vi "Testing Functional Test.vi"(7 "FrequencyCounter":refnum<visa-resource-name>, 8 "connection information":path, 9 "System Number":string, 10 "error in":errorcluster, 11 "Arduino":refnum<visa-resource-name>) -> (1 "Functional Test Data":string, 2 "error out":errorcluster, 3 "Arduino":refnum<visa-resource-name>)   [LabVIEW 2024]
uses:
  <vilib>/addons/database/Connection.llb/DB Tools Open Connec (Path).vi
  Agilent 532XX Series/Public/Configure/Measurement/Configure Measurement (Frequency).vi
  <vilib>/addons/database/_DB Variant To Data/Database Variant To Data.xnode
  <vilib>/addons/database/NI_Database_API.lvlib
  Agilent 532XX Series/Agilent 532XX Series.lvlib
panel:
  out "Command Array":string[](array[string])
  out "Upper Position":i32
  out "Lower Position":i32
  out "Functional Test Data Rack 2":string
  out "Functional Test Data Rack 1":string
  out "Lower Rack":dbl
  out "Upper Rack":dbl
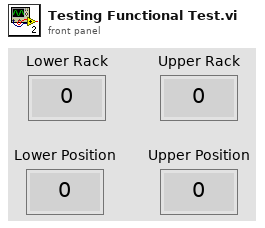
[diagram p1: front panel]
types:
  T1 = typedef "NI_Database_API.lvlib/Conn ObjectReference.ctl" = refnum<k1>
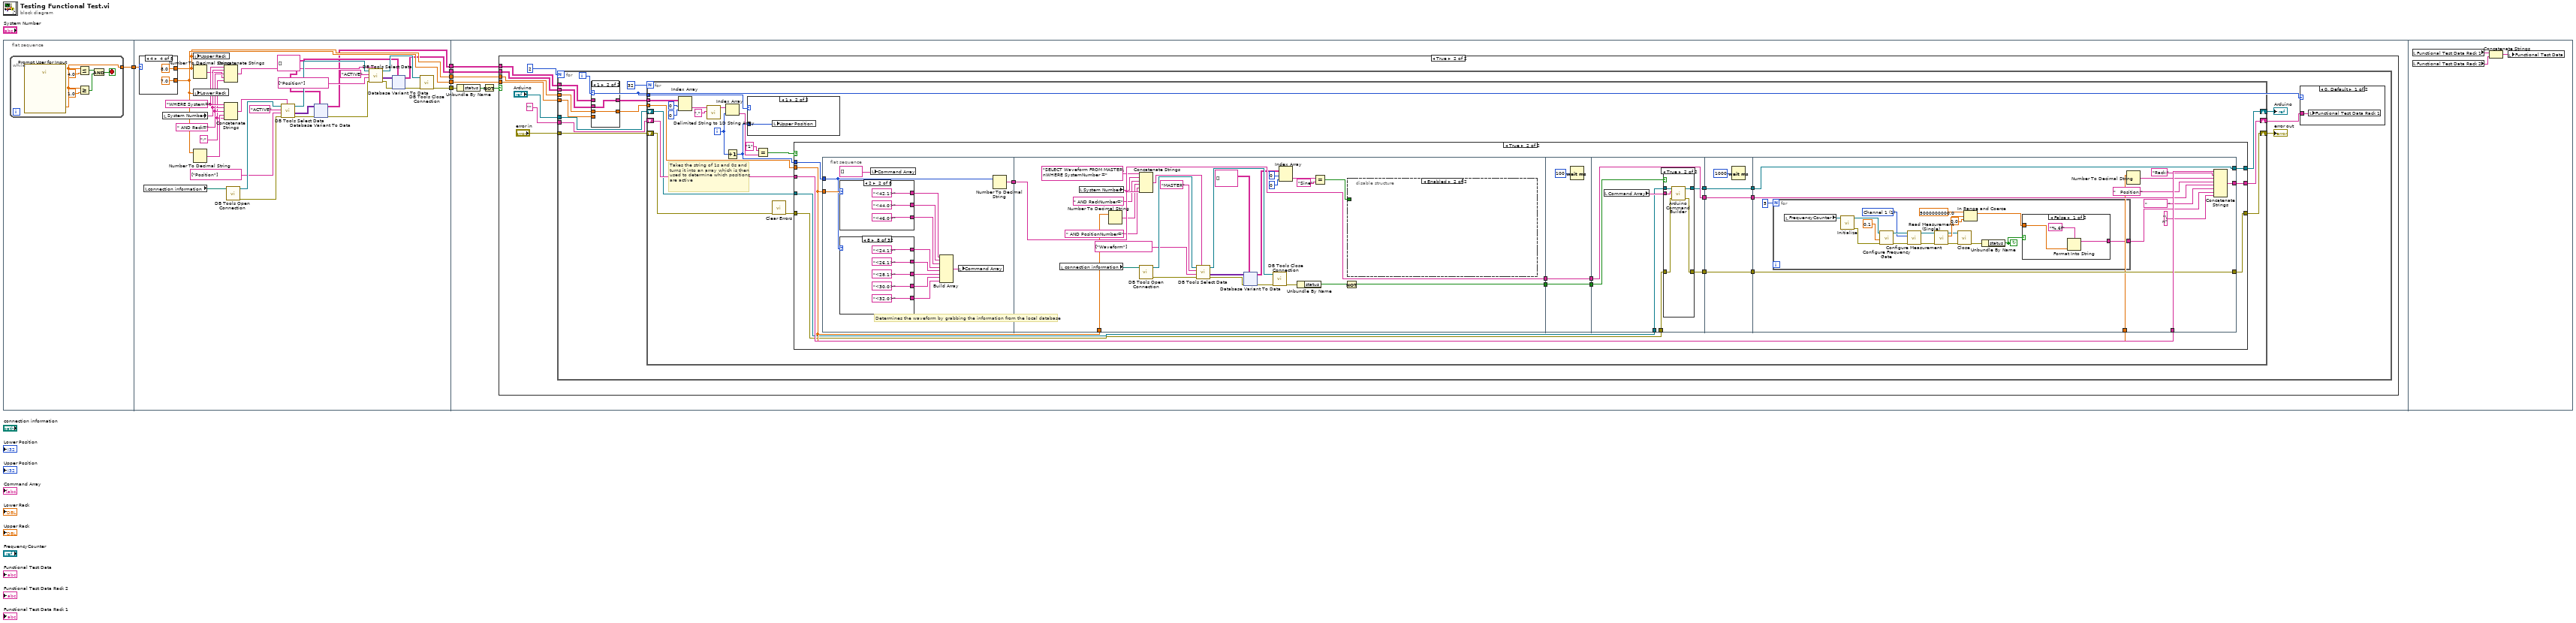
[diagram p0: block diagram]
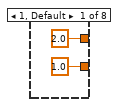
[diagram p2: hidden frame]
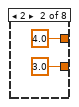
[diagram p3: hidden frame]
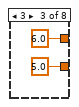
[diagram p4: hidden frame]
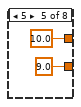
[diagram p5: hidden frame]
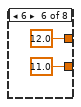
[diagram p6: hidden frame]
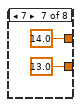
[diagram p7: hidden frame]
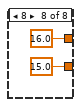
[diagram p8: hidden frame]
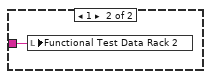
[diagram p10: hidden frame]
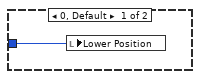
[diagram p12: hidden frame]
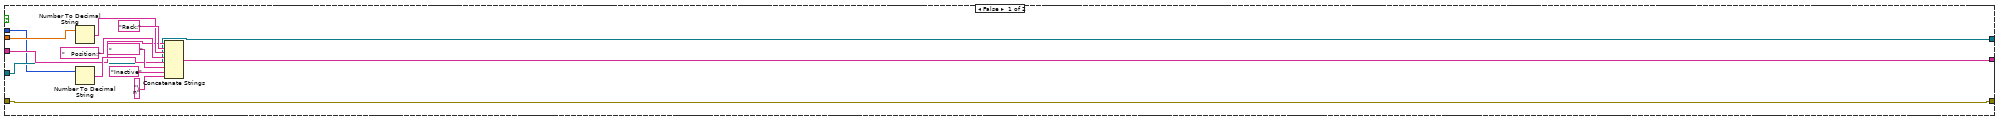
[diagram p13: hidden frame]
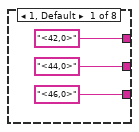
[diagram p14: hidden frame]
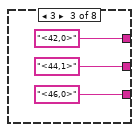
[diagram p15: hidden frame]
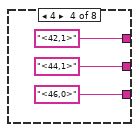
[diagram p16: hidden frame]
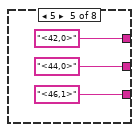
[diagram p17: hidden frame]
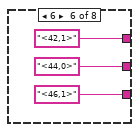
[diagram p18: hidden frame]
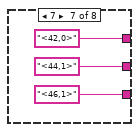
[diagram p19: hidden frame]
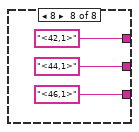
[diagram p20: hidden frame]
diagram:
  n1 = flat-sequence {
    tunnel: [w7] -> w2
    tunnel: [w16] -> w6
    tunnel: [w15] -> w5
    tunnel: [w36] -> w4
    tunnel: [w38] -> w3
    tunnel: w2 -> [w35]
    tunnel: [w30] -> w1
    tunnel: w3 -> [w153]
    tunnel: w4 -> [w154]
    tunnel: w5 -> [w151]
    tunnel: w6 -> [w152]
    tunnel: w1 -> [w148]
    frame #0 {
      n2 = while {
        tunnel: [w13] -> w7
        stop <- w10 stop-if-true
        n3 = call "Prompt User for Input"() -> ("Shelf Number"=w13:dbl)  [unwired: 17 in, 2 out]
        n4 = Less Or Equal?(x=w13, y=4.0) -> (x <= y?=w9:bool)
        n5 = Greater Or Equal?(x=w13, y=1.0) -> (x >= y?=w8:bool)
        n6 = And(x=w9, y=w8) -> (x .and. y?=w10:bool)
      }
    }
    frame #1 {
      w18 = string[][] []
      w41 = " AND Rack="
      w39 = ";" ("string")
      w42 = "WHERE System=" ("SQL Query")
      n7 = case shown="4" w35 {
        tunnel: [1.0 ("y") 3.0 ("y") 5.0 ("y") 7.0 ("y") 9.0 ("y") 11.0 ("y") 13.0 ("y") 15.0 ("y")] -> w38
        tunnel: [2.0 ("y") 4.0 ("y") 6.0 ("y") 8.0 ("y") 10.0 ("y") 12.0 ("y") 14.0 ("y") 16.0 ("y")] -> w36
        frame 1, Default {
        }
        frame 2 {
        }
        frame 3 {
        }
        frame 4 {
        }
        frame 5 {
        }
        frame 6 {
        }
        frame 7 {
        }
        frame 8 {
        }
      }
      n8 = local read "connection information"() -> (w14:path)
      n9 = local read "System Number"() -> (w40:string)
      n10 = local write "Upper Rack"(w36) -> ()
      n11 = Number To Decimal String(number=w36) -> (decimal integer string=w37:string)  [unwired: 1 in]
      n12 = local write "Lower Rack"(w38) -> ()
      n13 = Number To Decimal String(number=w38) -> (decimal integer string=w43:string)  [unwired: 1 in]
      n14 = Concatenate Strings(w42, w40, w41, w37, w39) -> (w21:string)
      n15 = Concatenate Strings(w42, w40, w41, w43, w39) -> (w20:string)
      n16 = call-poly <vilib>:"DB Tools Open Connection.vi"("connection information"=w14) -> ("error out"=w29:errorcluster, "connection reference"=w28:T1)  [unwired: 7 in]
      n17 = call <vilib>:"DB Tools Select Data.vi"("condition"=w20, "error in (no error)"=w29, "columns"=string[] ["Position"], "table"="ACTIVE", "connection reference"=w28) -> ("error out"=w34:errorcluster, "data"=w17:variant[][], "connection reference out"=w27:T1)  [unwired: 1 in]
      n18 = xnode "Database Variant To Data"("database variant"=w17, "error in (no error)"=w34, "type"=w18) -> ("data"=w16:string[][], "error out"=w33:errorcluster)
      n19 = call <vilib>:"DB Tools Select Data.vi"("condition"=w21, "error in (no error)"=w33, "columns"=string[] ["Position"], "table"="ACTIVE", "connection reference"=w27) -> ("error out"=w32:errorcluster, "data"=w19:variant[][], "connection reference out"=w26:T1)  [unwired: 1 in]
      n20 = xnode "Database Variant To Data"("database variant"=w19, "error in (no error)"=w32, "type"=w18) -> ("data"=w15:string[][], "error out"=w31:errorcluster)
      n21 = call <vilib>:"DB Tools Close Connection.vi"("error in (no error)"=w31, "connection reference"=w26) -> ("error out"=w30:errorcluster)  [unwired: 5 in]
    }
    frame #2 {
      n22 = Unbundle By Name(w148) -> ("status"=w150:bool)
      n23 = Not(x=w150) -> (.not. x?=w149:bool)
      n24 = case shown="True" w149 {
        tunnel: w154 -> [_ w158]
        tunnel: w153 -> [_ w157]
        tunnel: w152 -> [_ w156]
        tunnel: w151 -> [_ w155]
        frame False {
        }
        frame True {
          n25 = for {
            N: 2 -> [_]
            tunnel: "" -> [w176]
            tunnel: w156 -> [w172]
            tunnel: "error in" -> [w174]
            tunnel: "Arduino" -> [w173]
            tunnel: w155 -> [w171]
            tunnel: w158 -> [w169]
            tunnel: w157 -> [w168]
            i -> [w165]
            n26 = case shown="1" w165 {
              tunnel: w172 -> [w180 _]
              tunnel: w171 -> [_ w182]
              tunnel: [w180 w182] -> w170
              tunnel: w169 -> [_ w181]
              tunnel: w168 -> [w179 _]
              tunnel: [w179 w181] -> w167
              frame 0, Default {
              }
              frame 1 {
              }
            }
            n27 = for {
              N: 32 -> [_]
              shift-right: [w191] -> w166
              shift-left: w176 -> [w192]
              tunnel: w167 -> [w193]
              tunnel: w170 -> [w197]
              shift-right: [w189] -> w164
              shift-left: w173 -> [w184]
              shift-right: [w190] -> w163
              shift-left: w174 -> [w202]
              tunnel: w165 -> [w185]
              i -> [w187]
              # "Takes the string of 1s and 0s and turns it into an array which is then used to determine which positions are active"
              n28 = Index Array(array=w197, index (row)=0 ("disabled index (row)"), index (col)=0 ("disabled index (col)")) -> (element=w199:string)
              n29 = call <vilib>:"Delimited String to 1D String Array.vi"("delimiter"=",", "delimited string"=w199) -> ("string array"=w200:string[])  [unwired: 9 in]
              n30 = Index Array(array=w200, index=w187) -> (element=w201:string)
              n31 = Increment(x=w187) -> (x+1=w186:i32)
              n32 = case shown="1" w185 {
                tunnel: w186 -> [w203 w204]
                frame 0, Default {
                  n33 = local write "Lower Position"(w203) -> ()
                }
                frame 1 {
                  n34 = local write "Upper Position"(w204) -> ()
                }
              }
              n35 = Equal?(x="1", y=w201) -> (x = y?=w188:bool)
              n36 = call <vilib>:"Clear Errors.vi"("error in (no error)"=w202) -> ("error out"=w183:errorcluster)  [unwired: 5 in, 1 out]
              n37 = case shown="True" w188 {
                tunnel: w186 -> [w205 w236]
                tunnel: w193 -> [w208 w230]
                tunnel: w192 -> [w209 w235]
                tunnel: w184 -> [w206 w220]
                tunnel: w183 -> [w207 w225]
                tunnel: [w211 w234] -> w191
                tunnel: [w207 w233] -> w190
                tunnel: [w206 w232] -> w189
                frame False {
                  n38 = Number To Decimal String(number=w208) -> (decimal integer string=w216:string)  [unwired: 1 in]
                  n39 = Number To Decimal String(number=w205) -> (decimal integer string=w210:string)  [unwired: 1 in]
                  n40 = Concatenate Strings(w209, "Rack:" ("string"), w216, "   Position:" ("string"), w210, "              " ("string"), "Inactive" ("string"), "\n" ("string")) -> (w211:string)
                }
                frame True {
                  n41 = flat-sequence {
                    tunnel: [w249] -> w231
                    tunnel: w236 -> [w247]
                    tunnel: w230 -> [w248]
                    tunnel: w231 -> [w460]
                    tunnel: [w460] -> w229
                    tunnel: w230 -> [w452]
                    tunnel: [w447] -> w218
                    tunnel: w229 -> [w520]
                    tunnel: [w520] -> w228
                    tunnel: [w518] -> w219
                    tunnel: w218 -> [w518]
                    tunnel: w228 -> [w527]
                    tunnel: [w527] -> w227
                    tunnel: w225 -> [w525]
                    tunnel: [w524] -> w223
                    tunnel: [w523] -> w221
                    tunnel: w220 -> [w522]
                    tunnel: w219 -> [w521]
                    tunnel: w227 -> [w538]
                    tunnel: [w538] -> w226
                    tunnel: [w536] -> w224
                    tunnel: w223 -> [w536]
                    tunnel: [w535] -> w222
                    tunnel: w221 -> [w535]
                    tunnel: w235 -> [w551]
                    tunnel: w230 -> [w541]
                    tunnel: [w550] -> w234
                    tunnel: [w543] -> w233
                    tunnel: [w542] -> w232
                    tunnel: w226 -> [w549]
                    tunnel: w224 -> [w543]
                    tunnel: w222 -> [w542]
                    frame #0 {
                      # "Determines the waveform by grabbing the information from the local database"
                      n42 = case shown="2" w248 {
                        tunnel: ["<42,0>" ("string") "<42,1>" ("string") "<42,0>" ("string") "<42,1>" ("string") "<42,0>" ("string") "<42,1>" ("string") "<42,0>" ("string") "<42,1>" ("string")] -> w240
                        tunnel: ["<44,0>" ("string") "<44,0>" ("string") "<44,1>" ("string") "<44,1>" ("string") "<44,0>" ("string") "<44,0>" ("string") "<44,1>" ("string") "<44,1>" ("string")] -> w239
                        tunnel: ["<46,0>" ("string") "<46,0>" ("string") "<46,0>" ("string") "<46,0>" ("string") "<46,1>" ("string") "<46,1>" ("string") "<46,1>" ("string") "<46,1>" ("string")] -> w238
                        frame 1, Default {
                        }
                        frame 2 {
                        }
                        frame 3 {
                        }
                        frame 4 {
                        }
                        frame 5 {
                        }
                        frame 6 {
                        }
                        frame 7 {
                        }
                        frame 8 {
                        }
                      }
                      n43 = case shown="8" w247 {
                        tunnel: ["<32,0>" ("string") "<32,0>" ("string") "<32,0>" ("string") "<32,0>" ("string") "<32,0>" ("string") "<32,0>" ("string") "<32,0>" ("string") "<32,0>" ("string") "<32,0>" ("string") "<32,0>" ("string") "<32,0>" ("string") "<32,0>" ("string") "<32,0>" ("string") "<32,0>" ("string") "<32,0>" ("string") "<32,0>" ("string") "<32,1>" ("string") "<32,1>" ("string") "<32,1>" ("string") "<32,1>" ("string") "<32,1>" ("string") "<32,1>" ("string") "<32,1>" ("string") "<32,1>" ("string") "<32,1>" ("string") "<32,1>" ("string") "<32,1>" ("string") "<32,1>" ("string") "<32,1>" ("string") "<32,1>" ("string") "<32,1>" ("string") "<32,1>" ("string")] -> w242
                        tunnel: ["<30,0>" ("string") "<30,0>" ("string") "<30,0>" ("string") "<30,0>" ("string") "<30,0>" ("string") "<30,0>" ("string") "<30,0>" ("string") "<30,0>" ("string") "<30,1>" ("string") "<30,1>" ("string") "<30,1>" ("string") "<30,1>" ("string") "<30,1>" ("string") "<30,1>" ("string") "<30,1>" ("string") "<30,1>" ("string") "<30,0>" ("string") "<30,0>" ("string") "<30,0>" ("string") "<30,0>" ("string") "<30,0>" ("string") "<30,0>" ("string") "<30,0>" ("string") "<30,0>" ("string") "<30,1>" ("string") "<30,1>" ("string") "<30,1>" ("string") "<30,1>" ("string") "<30,1>" ("string") "<30,1>" ("string") "<30,1>" ("string") "<30,1>" ("string")] -> w243
                        tunnel: ["<28,0>" ("string") "<28,0>" ("string") "<28,0>" ("string") "<28,0>" ("string") "<28,1>" ("string") "<28,1>" ("string") "<28,1>" ("string") "<28,1>" ("string") "<28,0>" ("string") "<28,0>" ("string") "<28,0>" ("string") "<28,0>" ("string") "<28,1>" ("string") "<28,1>" ("string") "<28,1>" ("string") "<28,1>" ("string") "<28,0>" ("string") "<28,0>" ("string") "<28,0>" ("string") "<28,0>" ("string") "<28,1>" ("string") "<28,1>" ("string") "<28,1>" ("string") "<28,1>" ("string") "<28,0>" ("string") "<28,0>" ("string") "<28,0>" ("string") "<28,0>" ("string") "<28,1>" ("string") "<28,1>" ("string") "<28,1>" ("string") "<28,1>" ("string")] -> w244
                        tunnel: ["<26,0>" ("string") "<26,0>" ("string") "<26,1>" ("string") "<26,1>" ("string") "<26,0>" ("string") "<26,0>" ("string") "<26,1>" ("string") "<26,1>" ("string") "<26,0>" ("string") "<26,0>" ("string") "<26,1>" ("string") "<26,1>" ("string") "<26,0>" ("string") "<26,0>" ("string") "<26,1>" ("string") "<26,1>" ("string") "<26,0>" ("string") "<26,0>" ("string") "<26,1>" ("string") "<26,1>" ("string") "<26,0>" ("string") "<26,0>" ("string") "<26,1>" ("string") "<26,1>" ("string") "<26,0>" ("string") "<26,0>" ("string") "<26,1>" ("string") "<26,1>" ("string") "<26,0>" ("string") "<26,0>" ("string") "<26,1>" ("string") "<26,1>" ("string")] -> w245
                        tunnel: ["<24,0>" ("string") "<24,1>" ("string") "<24,0>" ("string") "<24,1>" ("string") "<24,0>" ("string") "<24,1>" ("string") "<24,0>" ("string") "<24,1>" ("string") "<24,0>" ("string") "<24,1>" ("string") "<24,0>" ("string") "<24,1>" ("string") "<24,0>" ("string") "<24,1>" ("string") "<24,0>" ("string") "<24,1>" ("string") "<24,0>" ("string") "<24,1>" ("string") "<24,0>" ("string") "<24,1>" ("string") "<24,0>" ("string") "<24,1>" ("string") "<24,0>" ("string") "<24,1>" ("string") "<24,0>" ("string") "<24,1>" ("string") "<24,0>" ("string") "<24,1>" ("string") "<24,0>" ("string") "<24,1>" ("string") "<24,0>" ("string") "<24,1>" ("string")] -> w246
                        frame 1, Default {
                        }
                        frame 2 {
                        }
                        frame 3 {
                        }
                        frame 4 {
                        }
                        frame 5 {
                        }
                        frame 6 {
                        }
                        frame 7 {
                        }
                        frame 8 {
                        }
                        frame 9 {
                        }
                        frame 10 {
                        }
                        frame 11 {
                        }
                        frame 12 {
                        }
                        frame 13 {
                        }
                        frame 14 {
                        }
                        frame 15 {
                        }
                        frame 16 {
                        }
                        frame 17 {
                        }
                        frame 18 {
                        }
                        frame 19 {
                        }
                        frame 20 {
                        }
                        frame 21 {
                        }
                        frame 22 {
                        }
                        frame 23 {
                        }
                        frame 24 {
                        }
                        frame 25 {
                        }
                        frame 26 {
                        }
                        frame 27 {
                        }
                        frame 28 {
                        }
                        frame 29 {
                        }
                        frame 30 {
                        }
                        frame 31 {
                        }
                        frame 32 {
                        }
                      }
                      n44 = local write "Command Array"(string[] [] ("Command Array")) -> ()
                      n45 = Build Array(w240, w239, w238, w246, w245, w244, w243, w242) -> (w241:string[])
                      n46 = local write "Command Array"(w241) -> ()
                      n47 = Number To Decimal String(number=w247) -> (decimal integer string=w249:string)  [unwired: 1 in]
                    }
                    frame #1 {
                      n48 = local read "connection information"() -> (w444:path)
                      n49 = local read "System Number"() -> (w457:string)
                      n50 = Number To Decimal String(number=w452) -> (decimal integer string=w458:string)  [unwired: 1 in]
                      n51 = Concatenate Strings("SELECT Waveform FROM MASTER\nWHERE SystemNumber =" ("SQL Query"), w457, " AND RackNumber=" ("string"), w458, " AND PositionNumber=" ("string"), w460) -> (w441:string)
                      n52 = call-poly <vilib>:"DB Tools Open Connection.vi"("connection information"=w444) -> ("error out"=w445:errorcluster, "connection reference"=w443:T1)  [unwired: 7 in]
                      n53 = call <vilib>:"DB Tools Select Data.vi"("condition"=w441, "error in (no error)"=w445, "columns"=string[] ["Waveform"], "table"="MASTER", "connection reference"=w443) -> ("error out"=w446:errorcluster, "data"=w435:variant[][], "connection reference out"=w439:T1)  [unwired: 1 in]
                      n54 = xnode "Database Variant To Data"("database variant"=w435, "error in (no error)"=w446, "type"=string[][] []) -> ("data"=w437:string[][], "error out"=w438:errorcluster)
                      n55 = call <vilib>:"DB Tools Close Connection.vi"("error in (no error)"=w438, "connection reference"=w439) -> ("error out"=w434:errorcluster)  [unwired: 5 in]
                      n56 = Index Array(array=w437, index (row)=0, index (col)=0) -> (element=w459:string)
                      n57 = Unbundle By Name(w434) -> ("status"=w448:bool)
                      n58 = Equal?(x=w459, y="Sine") -> (x = y?=w456:bool)
                      n59 = Not(x=w448) -> (.not. x?=w447:bool)
                      n60 = disable-structure shown="Enabled" {
                        disable-tunnel: w456 -> [w461 _]
                        frame Disabled {
                          n61 = case shown="True" w461 {
                            frame False {
                              n62 = flat-sequence {
                                frame #0 {
                                n63 = Send(0:0 ("bus"), 2:i16 3 ("address"), 5:"INP:COUP DC " ("data string")) -> ()  [unwired: 2 in, 3 out]
                                }
                                frame #1 {
                                n64 = Send(0:0 ("bus"), 2:i16 3 ("address"), 5:"INP:IMP 1.0E6" ("data string")) -> ()  [unwired: 2 in, 3 out]
                                }
                              }
                            }
                            frame True {
                              n65 = flat-sequence {
                                frame #0 {
                                n66 = Send(0:0 ("bus"), 2:i16 3 ("address"), 5:"INP:COUP AC " ("data string")) -> ()  [unwired: 2 in, 3 out]
                                }
                                frame #1 {
                                n67 = Send(0:0 ("bus"), 2:i16 3 ("address"), 5:"INP:IMP 50" ("data string")) -> ()  [unwired: 2 in, 3 out]
                                }
                              }
                            }
                          }
                        }
                        frame Enabled {
                        }
                      }
                    }
                    frame #2 {
                      n68 = Wait (ms)(milliseconds to wait=u32 100) -> ()  [unwired: 1 out]
                    }
                    frame #3 {
                      n69 = local read "Command Array"() -> (w526:string[])
                      n70 = case shown="True" w521 {
                        tunnel: w526 -> [_ w534]
                        tunnel: w525 -> [w528 w533]
                        tunnel: [w528 w532] -> w524
                        tunnel: [w529 w531] -> w523
                        tunnel: w522 -> [w529 w530]
                        frame False {
                        }
                        frame True {
                          n71 = call "Arduino Command Builder.vi"("error in"=w533, "Commands"=w534, "Arduino in"=w530) -> ("error out"=w532:errorcluster, "Arduino out"=w531:refnum<visa-resource-name>)  [unwired: 7 in]
                        }
                      }
                    }
                    frame #4 {
                      n72 = Wait (ms)(milliseconds to wait=u32 1000) -> ()  [unwired: 1 out]
                    }
                    frame #5 {
                      n73 = for {
                        N: 5 -> [_]
                        tunnel: [w552] -> w544
                        stop <- w553 continue-if-true
                        w557 = 1 items=["Channel 1"=1, "Channel 2"=2, "Channel 3"=3] ("Channel (1:Channel 1)")
                        n74 = local read "FrequencyCounter"() -> (w564:refnum<visa-resource-name>)
                        n75 = call "Initialize.vi"("VISA resource name"=w564) -> ("error out"=w559:errorcluster, "VISA resource name out"=w558:refnum<visa-resource-name>)  [unwired: 9 in]
                        n76 = call "Configure Frequency Gate.vi"("error in (no error)"=w559, "Time Resolution (0.1 s)"=0.1 ("number"), "VISA resource name"=w558) -> ("error out"=w568:errorcluster, "VISA resource name out"=w565:refnum<visa-resource-name>)  [unwired: 7 in]
                        n77 = call-poly "Configure Measurement.vi"("error in (no error)"=w568, "Channel (1:Channel 1)"=w557, "VISA resource name"=w565) -> ("error out"=w567:errorcluster, "VISA resource name out"=w566:refnum<visa-resource-name>)  [unwired: 2 in, 5 out]
                        n78 = call "Read Measurement (Single).vi"("error in (no error)"=w567, "VISA resource name"=w566) -> ("error out"=w561:errorcluster, "Measurement"=w562:dbl, "VISA resource name out"=w560:refnum<visa-resource-name>)  [unwired: 7 in]
                        n79 = call "Close.vi"("error in (no error)"=w561, "VISA resource name"=w560) -> ("error out"=w563:errorcluster)  [unwired: 9 in]
                        n80 = In Range and Coerce(upper limit=5000000000.0, x=w562, lower limit=0.0) -> (coerced(x)=w569:dbl)  [unwired: 1 out]
                        n81 = Unbundle By Name(w563) -> ("status"=w553:bool)
                        n82 = case shown="False" w553 {
                          tunnel: [w570 "N/A"] -> w552
                          tunnel: w569 -> [w571 _]
                          frame False {
                            n83 = Format Into String(format string="%.6f", w571) -> (resulting string=w570:string)  [unwired: 2 in, 1 out]
                          }
                          frame True {
                            n84 = local read "FrequencyCounter"() -> (w574:refnum<visa-resource-name>)
                            n85 = VISA Clear(VISA resource name=w574) -> ()  [unwired: 1 in, 2 out]
                          }
                        }
                      }
                      n86 = Number To Decimal String(number=w541) -> (decimal integer string=w547:string)  [unwired: 1 in]
                      n87 = Concatenate Strings(w551, "Rack:" ("string"), w547, "   Position:" ("string"), w549, "              " ("string"), w544, "\n" ("string")) -> (w550:string)
                    }
                  }
                }
              }
            }
            "Arduino" <- w164
            "error out" <- w163
            n88 = case shown="0, Default" w165 {
              tunnel: w166 -> [w177 w178]
              frame 0, Default {
                n89 = local write "Functional Test Data Rack 1"(w177) -> ()
              }
              frame 1 {
                n90 = local write "Functional Test Data Rack 2"(w178) -> ()
              }
            }
          }
        }
      }
    }
    frame #3 {
      n91 = local read "Functional Test Data Rack 1"() -> (w576:string)
      n92 = local read "Functional Test Data Rack 2"() -> (w577:string)
      n93 = Concatenate Strings(w576, w577) -> (w575:string)
      n94 = local write "Functional Test Data"(w575) -> ()
    }
  }
